vi "CIC_5decimate_1cycle.vi"(7 "reset":bool, 8 "valid in":bool, 11 "Data in":fxp<+/-,32,14>) -> (0 "valid out":bool, 3 "Data out":fxp<+/-,32,14>)   [LabVIEW 2018]
uses:
  <vilib>/rvi/FXPMathLib/FxpConvert/subVIs/nifxpmath_Convert_SimConfig.ctl
  <vilib>/fxp/LVFixedPointQuantizationPolicyTypeDef.ctl
  <vilib>/fxp/LVFixedPointOverflowPolicyTypeDef.ctl
  <vilib>/rvi/IPIntegrationNode/IPINode_Typedef/niFpgaIPINodeSupportedFamilies.ctl
  <vilib>/rvi/FXPMathLib/FxpConvert/simVIs/DllFxpConvertTemp_sub.vi
  <vilib>/rvi/IPIntegrationNode/IPINode_Utilities/niFpgaIPINodeSimCore.vi
  <vilib>/rvi/FXPMathLib/FxpInterpret/XNode/nifxpmath_Interpret.xnode
  <vilib>/rvi/FXPMathLib/FxpMul/XNode/nifxpmath_Multiplier.xnode
  <vilib>/rvi/FXPMathLib/FxpConvert/XNode/nifxpmath_Convert.xnode
  <vilib>/rvi/XilinxIP/XIPIN_XNode/niFpgaXIPIN.xnode
  Xilinx/CIC_5decimate_1cycle/CIC 5Decimate 1Cycle/xsim.dir/CIC_5Decimate_1Cycle_B9E366AD7870487A8CEE328F0D9947C8/xsimk_B9E366AD7870487A8CEE328F0D9947C8.dll
  <vilib>/rvi/IPIntegrationNode/IPINode_Xnode/niFpgaIPINode.xnode
  <vilib>/rvi/FXPMathLib/sim/FxpSim.dll
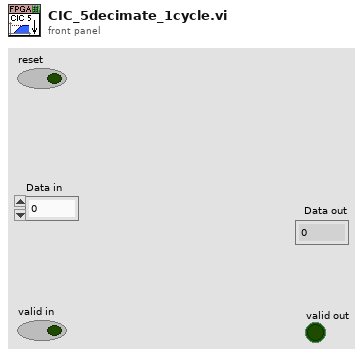
[diagram p1: front panel]
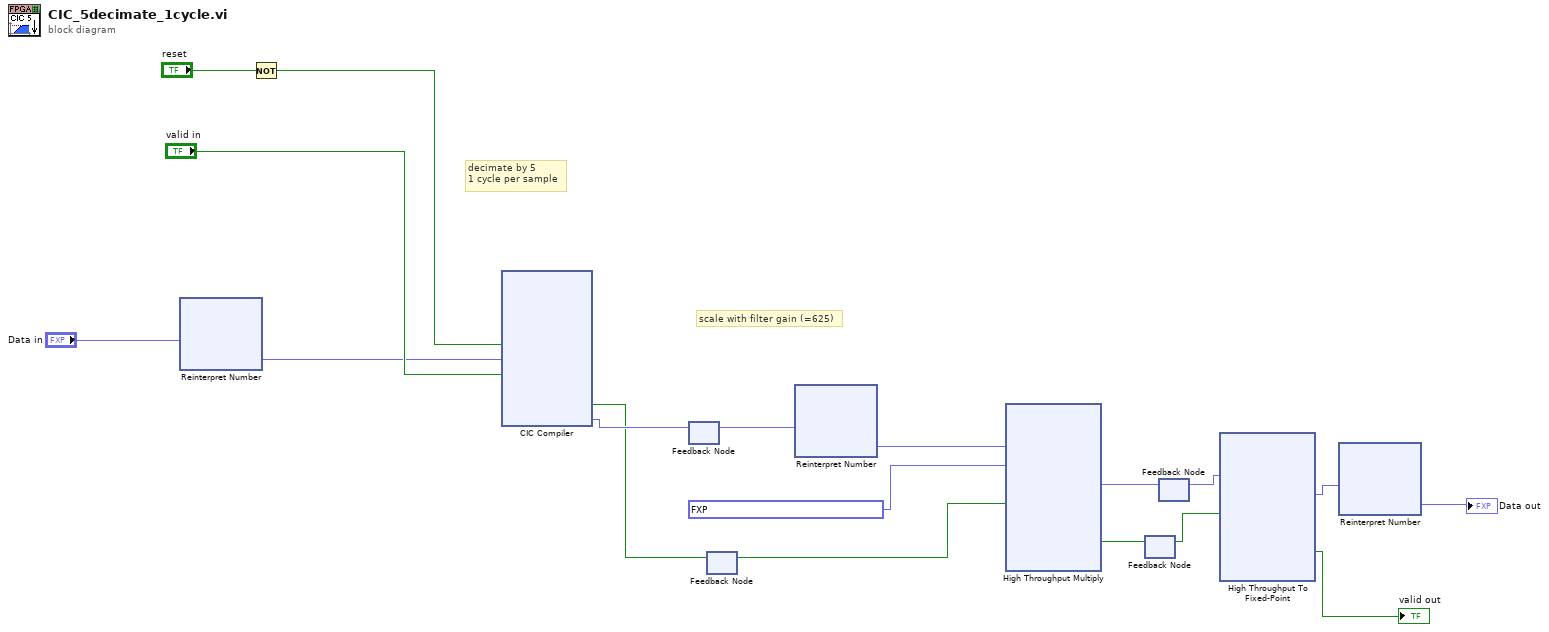
[diagram p0: block diagram]
diagram:
  # "decimate by 5\n1 cycle per sample"
  # "scale with filter gain (=625)"
  n1 = xnode "Reinterpret Number"("x"="Data in") -> ("y"=w14:fxp<+,32,32>)
  n2 = Not(x="reset") -> (.not. x?=w16:bool)
  n3 = xnode ("CIC Compiler")("aresetn"=w16, "s_axis_data_tdata"=w14, "s_axis_data_tvalid"="valid in") -> ("m_axis_data_tvalid"=w9:bool, "m_axis_data_tdata"=w13:fxp<+,48,48>)  [unwired: 1 in, 1 out]
  n4 = feedback-in #1(w13) -> ()
  n5 = feedback #1() -> (w12:fxp<+,48,48>)  [unwired: 1 in]
  n6 = feedback #2() -> (w8:bool)  [unwired: 1 in]
  n7 = feedback-in #2(w9) -> ()
  n8 = xnode "Reinterpret Number"("x"=w12) -> ("y"=w11:fxp<+/-,48,48>)
  n9 = xnode ("High Throughput Multiply")("x"=w11, "y"=fxp<+/-,32,1> 0.001600000075995922, "input valid"=w8) -> ("x*y"=w6:fxp<+/-,64,49>, "output valid"=w7:bool)  [unwired: 1 in, 1 out]
  n10 = feedback #3() -> (w3:bool)  [unwired: 1 in]
  n11 = feedback-in #3(w7) -> ()
  n12 = feedback #4() -> (w4:fxp<+/-,64,49>)  [unwired: 1 in]
  n13 = feedback-in #4(w6) -> ()
  n14 = xnode "High Throughput To Fixed-Point"("x"=w4, "input valid"=w3) -> ("y"=w2:fxp<+/-,32,32>, "output valid"=→"valid out":bool)  [unwired: 1 in, 1 out]
  n15 = xnode "Reinterpret Number"("x"=w2) -> ("y"=→"Data out":fxp<+/-,32,14>)
